vi "StageMoved.vi"(8 "error in (no error)":errorcluster, 10 "Home?":bool=TRUE, 11 "SPIController in":refnum<class "SPIController.lvclass">) -> (0 "error out":errorcluster, 3 "SPIController out":refnum<class "SPIController.lvclass">)   [LabVIEW 2023, in "SPIController.lvlib" / "SPIController.lvclass"]
uses:
  SPIController.lvclass
  SPIController.lvclass/SPIController.ctl
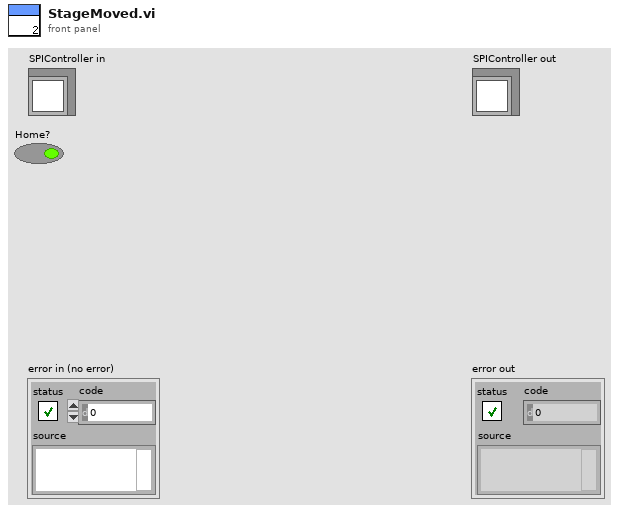
[diagram p1: front panel]
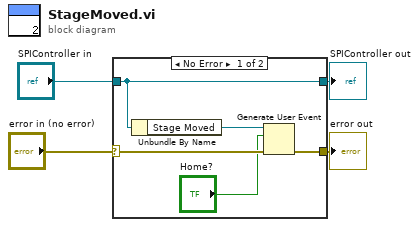
[diagram p0: block diagram]
diagram:
  n1 = case shown="No Error" "error in (no error)" {
    selector: "error in (no error)" -> [w8 w11]
    tunnel: [w7 w11] -> w3
    tunnel: [w9 w10] -> w1
    tunnel: "SPIController in" -> [w9 w10]
    frame No Error {
      n2 = Unbundle By Name(w9) -> ("Stage Moved"=w6:refnum<user-event>)
      n3 = Generate User Event(user event=w6, event data cluster="Home?", error in=w8) -> (error out=w7:errorcluster)  [unwired: 1 in, 1 out]
    }
    frame Error {
    }
  }
  "error out" <- w3
  "SPIController out" <- w1
